vi "oa_Scaled Window (N Channels).vi"(0 "resampled signals":cluster{"r0":dbl, "dr":dbl, "Y":dbl[]}[](array[cluster]) {"r0" format="%.2p"; "dr" format="%.2p"; "Y" format="%.2f"}, 1 "processing control in":T1(ring), 7 "spectrum settings":cluster{"window type":u32, "block size":i32}={"window type"=1, "block size"=400} {"block size" min=2; "window type" items=["None"=0, "Hanning"=1, "Hamming"=2, "Blackman-Harris"=3, "Exact Blackman"=4, "Blackman"=5, "Flat Top"=6, "4 Term B-Harris"=7, "7 Term B-Harris"=8, "Low Sidelobe"=9, "Gaussian"=62]}, 11 "error in":errorcluster) -> (3 "dup processing control":T1(ring), 4 "Y":dbl[][][](array[numeric]), 6 "new spectrum available?":bool, 8 "spectrum settings out":cluster{"window type":u32, "block size":i32}={"window type"=1, "block size"=400} {"block size" min=2; "window type" items=["None"=0, "Hanning"=1, "Hamming"=2, "Blackman-Harris"=3, "Exact Blackman"=4, "Blackman"=5, "Flat Top"=6, "4 Term B-Harris"=7, "7 Term B-Harris"=8, "Low Sidelobe"=9, "Gaussian"=62]}, 15 "error out":errorcluster)   [LabVIEW 2017, in "SoundVib_Resampling.lvlib"]
uses:
  <vilib>/addons/Sound and Vibration/Order Analysis/Resample Order Tracking/SoundVib_Resampling.lvlib
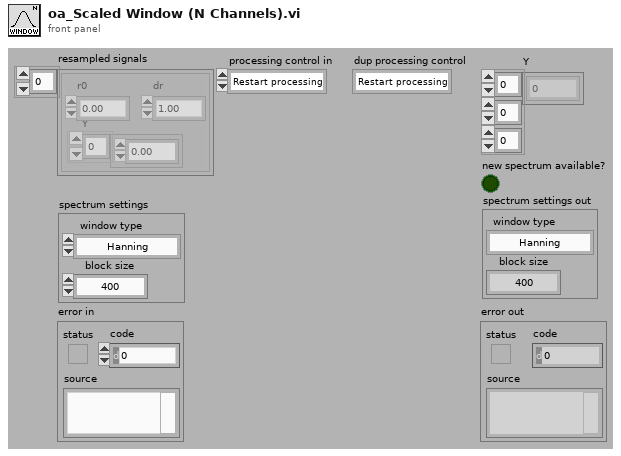
[diagram p1: front panel]
types:
  T1 = enum16{"Restart processing", "Continue processing", "Skip processing"}
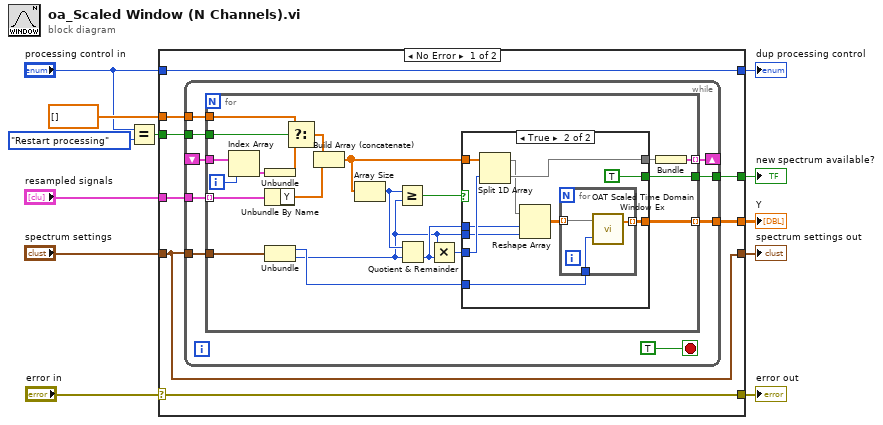
[diagram p0: block diagram]
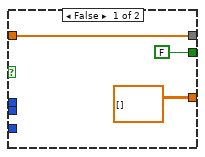
[diagram p2: hidden frame]
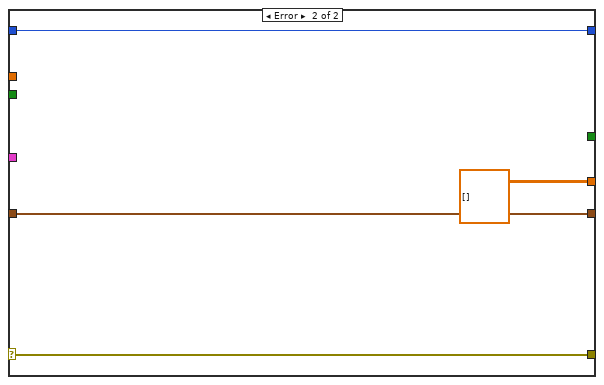
[diagram p3: hidden frame]
diagram:
  n1 = Equal?(x="processing control in", y=T1."Restart processing" ("processing control in")) -> (x = y?=w11:bool)
  n2 = case shown="No Error" "error in" {
    selector: "error in" -> [w20 w70]
    tunnel: [w20 w70] -> w3
    tunnel: "resampled signals" -> [w19 _]
    tunnel: "spectrum settings" -> [w18 w69]
    tunnel: [w18 w69] -> w5
    tunnel: [w17 dbl[][][] [] ("y")] -> w2
    tunnel: "processing control in" -> [w16 w67]
    tunnel: [w16 w67] -> w4
    tunnel: w11 -> [w15 _]
    tunnel: dbl[] [] ("t") -> [w14 _]
    tunnel: [w13 _] -> w1
    frame No Error {
      n3 = while {
        tunnel: w19 -> [w29]
        tunnel: w18 -> [w28]
        tunnel: [w27] -> w17
        tunnel: w15 -> [w26]
        tunnel: w14 -> [w25]
        shift-right: [w24] -> _
        shift-left: _ -> [w22]
        tunnel: [w21] -> w13
        stop <- TRUE stop-if-true
        n4 = for {
          tunnel: w29 -> [w50] mode=indexing
          tunnel: w28 -> [w49]
          tunnel: [w48] -> w27 mode=indexing
          tunnel: w26 -> [w47]
          tunnel: w25 -> [w46]
          tunnel: [w36] -> w24 mode=indexing
          tunnel: w22 -> [w35]
          tunnel: [w30] -> w21
          i -> [w34]
          n5 = Index Array(array=w35, index=w34) -> (element=w33:cluster{dbl[]})
          n6 = Unbundle(w33) -> (w32:dbl[])
          n7 = Unbundle By Name(w50) -> ("Y"=w45:dbl[])
          n8 = Unbundle(w49) -> ("window type"=w38:u32, "block size"=w31:i32)
          n9 = Select(t=w46, s=w47, f=w32) -> (s? t:f=w39:dbl[])
          n10 = Build Array (concatenate)(w39, w45) -> (w43:dbl[])
          n11 = Array Size(array=w43) -> (size(s)=w42:i32)
          n12 = Greater Or Equal?(x=w42, y=w31) -> (x >= y?=w44:bool)
          n13 = Quotient & Remainder(x=w42, y=w31) -> (floor(x/y)=w40:i32)  [unwired: 1 out]
          n14 = Multiply(x=w31, y=w40) -> (x*y=w41:i32)
          n15 = case shown="True" w44 {
            tunnel: w43 -> [w53 w63]
            tunnel: [w53 w61] -> w37
            tunnel: w41 -> [_ w62]
            tunnel: w40 -> [_ w59]
            tunnel: [dbl[][] [] w57] -> w48
            tunnel: w31 -> [_ w58]
            tunnel: w38 -> [_ w55]
            tunnel: [FALSE TRUE] -> w30
            frame False {
            }
            frame True {
              n16 = Split 1D Array(array=w63, index=w62) -> (first subarray=w60:dbl[], second subarray=w61:dbl[])
              n17 = Reshape Array(w60, w59, w58) -> (w56:dbl[][])
              n18 = for {
                tunnel: w56 -> [w66] mode=indexing
                tunnel: w55 -> [w65]
                tunnel: [w64] -> w57 mode=indexing
                n19 = call <vilib>:"OAT Scaled Time Domain Window Ex.vi"("window type"=w65, "X"=w66) -> ("y"=w64:dbl[])  [unwired: 1 out]
              }
            }
          }
          n20 = Bundle(w37) -> (w36:cluster{dbl[]})  [unwired: 1 in]
        }
      }
    }
    frame Error {
    }
  }
  "error out" <- w3
  "spectrum settings out" <- w5
  "dup processing control" <- w4
  "Y" <- w2
  "new spectrum available?" <- w1
